vi "X_2500_X5.vi"(0 "x0":dbl format="%#_13g", 5 "x1":dbl format="%#_13g", 7 "x2":dbl format="%#_13g", 9 "x3":dbl format="%#_13g", 11 "x4":dbl format="%#_13g", 12 "e":dbl format="%#_13g") -> (8 "X5out":dbl)   [LabVIEW 2019]
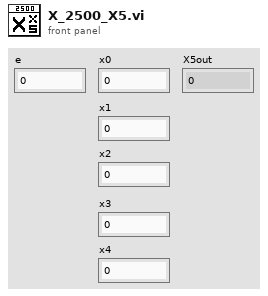
[diagram p1: front panel]
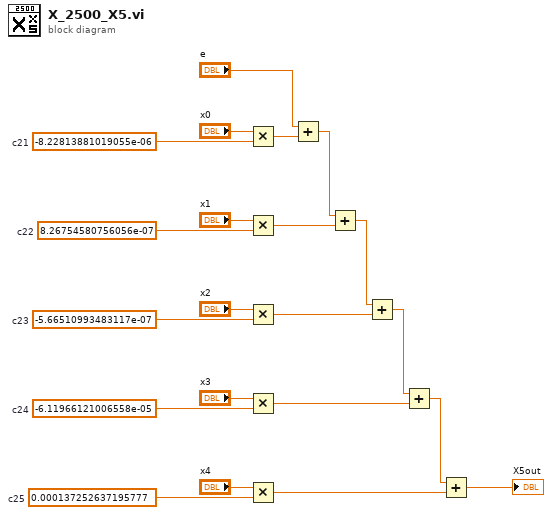
[diagram p0: block diagram]
diagram:
  w16 = -8.22813881019055e-06  # c21
  w14 = -5.66510993483117e-07  # c23
  w12 = 0.000137252637195777  # c25
  w13 = -6.11966121006558e-05  # c24
  w15 = 8.26754580756056e-07  # c22
  n1 = Multiply(x="x0", y=w16) -> (x*y=w3:dbl)
  n2 = Multiply(x="x1", y=w15) -> (x*y=w4:dbl)
  n3 = Multiply(x="x2", y=w14) -> (x*y=w5:dbl)
  n4 = Multiply(x="x3", y=w13) -> (x*y=w6:dbl)
  n5 = Multiply(x="x4", y=w12) -> (x*y=w7:dbl)
  n6 = Add(x="e", y=w3) -> (x+y=w11:dbl)
  n7 = Add(x=w11, y=w4) -> (x+y=w9:dbl)
  n8 = Add(x=w9, y=w5) -> (x+y=w10:dbl)
  n9 = Add(x=w10, y=w6) -> (x+y=w8:dbl)
  n10 = Add(x=w8, y=w7) -> (x+y=→"X5out":dbl)
